vi "Decode Default PDOs.vi"(1 "PDO 4":u8[](array[numeric]), 2 "PDO 3":u8[](array[numeric]), 3 "PDO 2":u8[](array[numeric]), 4 "PDO 1":u8[](array[numeric])) -> (0 "Decoded PDO":T1 {"Status word" format="%b"})   [LabVIEW 2016]
uses:
  Default PDO conf.ctl
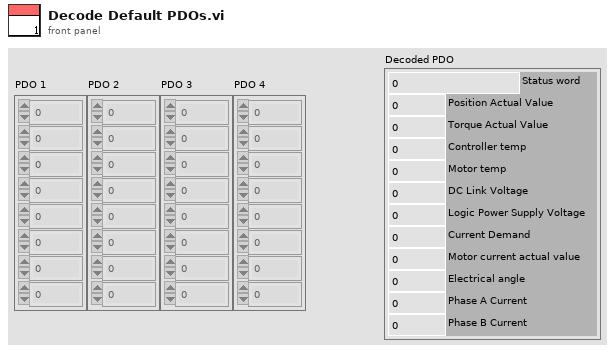
[diagram p1: front panel]
types:
  T1 = typedef "Default PDO conf.ctl" = cluster{"Status word":u16, "Position Actual Value":u32, "Torque Actual Value":u16, "Logic Power Supply Voltage":u16, "Current Demand":i32, "Controller temp":u8, "Motor temp":u8, "DC Link Voltage":u16, "Motor current actual value":u16, "Electrical angle":u16, "Phase A Current":u16, "Phase B Current":u16}
  T2 = cluster{"Status word":u16, "Position Actual Value":u32, "Torque Actual Value":u16, "Logic Power Supply Voltage":u16, "Current Demand":i32, "Controller temp":u8, "Motor temp":u8, "DC Link Voltage":u16, "Motor current actual value":u16, "Electrical angle":u16, "Phase A Current":u16, "Phase B Current":u16}
  T3 = cluster{"PDO 3[0]":u8, "PDO 3[1]":u8, "PDO 3[2]":u8, "PDO 3[3]":u8, "PDO 3[4]":u8, "PDO 3[5]":u8, "PDO 3[6]":u8, "PDO 3[7]":u8, "PDO 3[8]":u8}
  T4 = cluster{"PDO 2[0]":u8, "PDO 2[1]":u8, "PDO 2[2]":u8, "PDO 2[3]":u8, "PDO 2[4]":u8, "PDO 2[5]":u8, "PDO 2[6]":u8, "PDO 2[7]":u8, "PDO 2[8]":u8}
  T5 = cluster{"PDO 1[0]":u8, "PDO 1[1]":u8, "PDO 1[2]":u8, "PDO 1[3]":u8, "PDO 1[4]":u8, "PDO 1[5]":u8, "PDO 1[6]":u8, "PDO 1[7]":u8, "PDO 1[8]":u8}
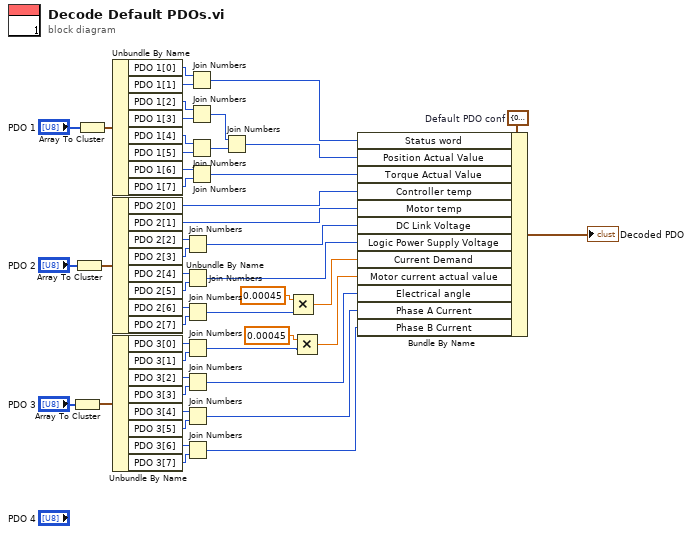
[diagram p0: block diagram]
diagram:
  w44 = T2 {"Status word"=0, "Position Actual Value"=0, "Torque Actual Value"=0, "Logic Power Supply Voltage"=0, "Current Demand"=0, "Controller temp"=0, "Motor temp"=0, "DC Link Voltage"=0, "Motor current actual value"=0, "Electrical angle"=0, "Phase A Current"=0, "Phase B Current"=0}  # Default PDO conf
  n1 = Array To Cluster(array="PDO 3") -> (cluster=w20:T3)
  n2 = Array To Cluster(array="PDO 2") -> (cluster=w32:T4)
  n3 = Array To Cluster(array="PDO 1") -> (cluster=w47:T5)
  n4 = Unbundle By Name(w47) -> ("PDO 1[0]"=w46:u8, "PDO 1[1]"=w45:u8, "PDO 1[2]"=w42:u8, "PDO 1[3]"=w41:u8, "PDO 1[4]"=w40:u8, "PDO 1[5]"=w39:u8, "PDO 1[6]"=w35:u8, "PDO 1[7]"=w34:u8)
  n5 = Unbundle By Name(w32) -> ("PDO 2[0]"=w30:u8, "PDO 2[1]"=w29:u8, "PDO 2[2]"=w28:u8, "PDO 2[3]"=w27:u8, "PDO 2[4]"=w25:u8, "PDO 2[5]"=w24:u8, "PDO 2[6]"=w22:u8, "PDO 2[7]"=w21:u8)
  n6 = Unbundle By Name(w20) -> ("PDO 3[0]"=w18:u8, "PDO 3[1]"=w17:u8, "PDO 3[2]"=w16:u8, "PDO 3[3]"=w15:u8, "PDO 3[4]"=w14:u8, "PDO 3[5]"=w13:u8, "PDO 3[6]"=w12:u8, "PDO 3[7]"=w11:u8)
  n7 = Join Numbers(hi=w28, lo=w27) -> ((hi.lo)=w26:u16)
  n8 = Join Numbers(hi=w25, lo=w24) -> ((hi.lo)=w23:u16)
  n9 = Join Numbers(hi=w22, lo=w21) -> ((hi.lo)=w4:u16)
  n10 = Join Numbers(hi=w18, lo=w17) -> ((hi.lo)=w2:u16)
  n11 = Join Numbers(hi=w16, lo=w15) -> ((hi.lo)=w10:u16)
  n12 = Join Numbers(hi=w14, lo=w13) -> ((hi.lo)=w9:u16)
  n13 = Join Numbers(hi=w12, lo=w11) -> ((hi.lo)=w8:u16)
  n14 = Join Numbers(hi=w46, lo=w45) -> ((hi.lo)=w43:u16)
  n15 = Join Numbers(hi=w42, lo=w41) -> ((hi.lo)=w37:u16)
  n16 = Join Numbers(hi=w40, lo=w39) -> ((hi.lo)=w38:u16)
  n17 = Join Numbers(hi=w35, lo=w34) -> ((hi.lo)=w33:u16)
  n18 = Join Numbers(hi=w37, lo=w38) -> ((hi.lo)=w36:u32)
  n19 = Multiply(x=0.00045, y=w4) -> (x*y=w3:dbl)
  n20 = Multiply(x=0.00045, y=w2) -> (x*y=w1:dbl)
  n21 = Bundle By Name(cluster=w44, "Status word"=w43, "Position Actual Value"=w36, "Torque Actual Value"=w33, "Controller temp"=w30, "Motor temp"=w29, "DC Link Voltage"=w26, "Logic Power Supply Voltage"=w23, "Current Demand"=w3, "Motor current actual value"=w1, "Electrical angle"=w10, "Phase A Current"=w9, "Phase B Current"=w8) -> (→"Decoded PDO":T2)
